vi "Configure Buffer.vi"(6 "Enable Buffer Statistics (0: Disable)":bool, 8 "error in (no error)":errorcluster, 9 "Buffer Source (0: None)":i32(ring) items=["None", "Measurements", "Math Calculation"], 10 "Buffer Size (2)":i32=2, 11 "VISA resource name":refnum<visa-resource-name>) -> (0 "error out":errorcluster, 3 "VISA resource name out":refnum<visa-resource-name>)   [LabVIEW 2022 SP3, in "Keithley 2182.lvlib"]
doc: "Configures the instrument's data bufffer which stores readings from a selected source."
uses:
  <instrlib>/Keithley 2182/Keithley 2182.lvlib
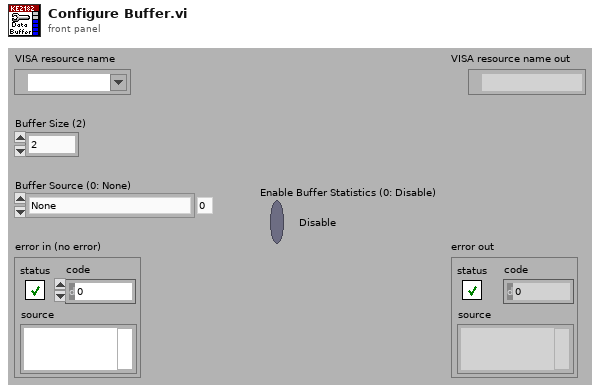
[diagram p1: front panel]
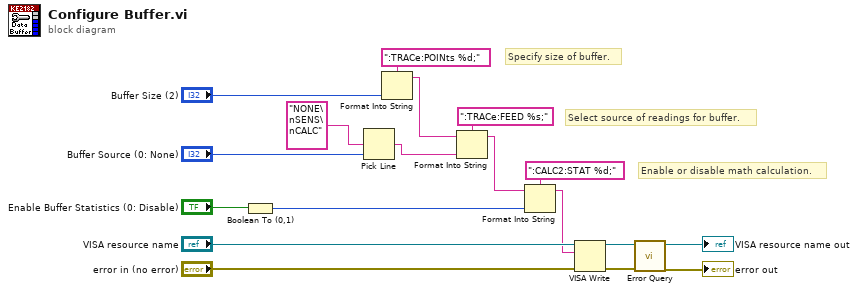
[diagram p0: block diagram]
diagram:
  # "Enable or disable math calculation."
  # "Select source of readings for buffer."
  # "Specify size of buffer."
  n1 = Boolean To (0,1)(Boolean="Enable Buffer Statistics (0: Disable)") -> (0, 1=w3:i16)
  n2 = Pick Line(multi-line string="NONE\nSENS\nCALC", line index="Buffer Source (0: None)") -> (output string=w8:string)  [unwired: 1 in]
  n3 = Format Into String(format string=":TRACe:POINts %d;", "Buffer Size (2)") -> (resulting string=w16:string)  [unwired: 2 in, 1 out]
  n4 = Format Into String(format string=":TRACe:FEED %s;", initial string=w16, w8) -> (resulting string=w1:string)  [unwired: 1 in, 1 out]
  n5 = Format Into String(format string=":CALC2:STAT %d;", initial string=w1, w3) -> (resulting string=w2:string)  [unwired: 1 in, 1 out]
  n6 = VISA Write(VISA resource name="VISA resource name", write buffer=w2, error in (no error)="error in (no error)") -> (VISA resource name out=w12:refnum<visa-resource-name>, error out=w11:errorcluster)  [unwired: 1 out]
  n7 = call <instrlib>:"Error Query.vi"("error in (no error)"=w11, "VISA resource name"=w12) -> ("error out"=→"error out":errorcluster, "VISA resource name out"=→"VISA resource name out":refnum<visa-resource-name>)  [unwired: 6 in, 2 out]
